vi "ReadWheelVelocity.vi"(8 "error in":errorcluster, 10 "Robot Configuration":T1={"wheel parameters"={"wheel radius"=0.05, "gear ratio"=1.0, "forward rotation direction"=0}, "wheel separation"=0.19, "Encoder Pulse Per Rev"=1856.0, "Update Period (sec)"=0.02, "Initial posture frame"=[0.0, 0.0, 0.0]} {"wheel parameters"."forward rotation direction" items=["Clockwise", "Counterclockwise"]}, 11 "Motor Ref":T4) -> (0 "error out":errorcluster, 2 "Wheel Velocity":T17, 3 "Motor Ref":T4)   [LabVIEW 2016]
uses:
  MotorObject.ctl
  <vilib>/myRIO/Instrument Drivers/Onboard IO/PWM/typedefs/PWM Reference.ctl
  <vilib>/myRIO/Common/Instrument Driver Framework/Utilities/typedefs/myRIO Generic Hardware Reference.ctl
  <vilib>/myRIO/Common/Instrument Driver Framework/Utilities/typedefs/Hardware Version Enum.ctl
  <vilib>/myRIO/Common/Instrument Driver Framework/Utilities/typedefs/myRIO v1.0 Reference.ctl
  <vilib>/myRIO/Common/Instrument Driver Framework/Utilities/typedefs/Generic FPGA Reference.ctl
  <vilib>/myRIO/Common/Instrument Driver Framework/myRIO v1.0/PWM/typedefs/PWM Channels Enum.ctl
  <vilib>/myRIO/Instrument Drivers/Onboard IO/PWM/typedefs/PWM Configuration.ctl
  <vilib>/myRIO/Instrument Drivers/Onboard IO/DIO/typedefs/DIO Reference.ctl
  <vilib>/myRIO/Common/Instrument Driver Framework/myRIO v1.0/DIO/typedefs/DIO Channels List.ctl
  <vilib>/myRIO/Common/Instrument Driver Framework/myRIO v1.0/DIO/typedefs/DIO Channels Enum.ctl
  <vilib>/myRIO/Instrument Drivers/Onboard IO/Encoder/typedefs/Encoder Reference.ctl
  <vilib>/myRIO/Common/Instrument Driver Framework/myRIO v1.0/Encoder/typedefs/Encoder Channels Enum.ctl
  Configurations.ctl
  <vilib>/robotics/Steering/Wheel/Wheel Parameters.ctl
  <vilib>/robotics/Steering/Wheel/Rotation Direction.ctl
  <vilib>/myRIO/Common/Instrument Driver Framework/myRIO v1.0/Encoder/vis/myRIO v1.0 Read Encoder.vi
  <vilib>/myRIO/Common/Instrument Driver Framework/roboRIO v1.0/Encoder/vis/roboRIO v1.0 Read Encoder.vi
  <vilib>/Utility/error.llb/Error Cluster From Error Code.vi
  <vilib>/myRIO/Instrument Drivers/Onboard IO/Encoder/Encoder.lvlib
  <vilib>/myRIO/Instrument Drivers/Onboard IO/DIO/DIO.lvlib
  <vilib>/myRIO/Instrument Drivers/Onboard IO/PWM/PWM.lvlib
  <vilib>/robotics/Steering/Wheel/NI_Robotics_Wheel.lvclass
panel:
  in  "Ref Cluster":T17
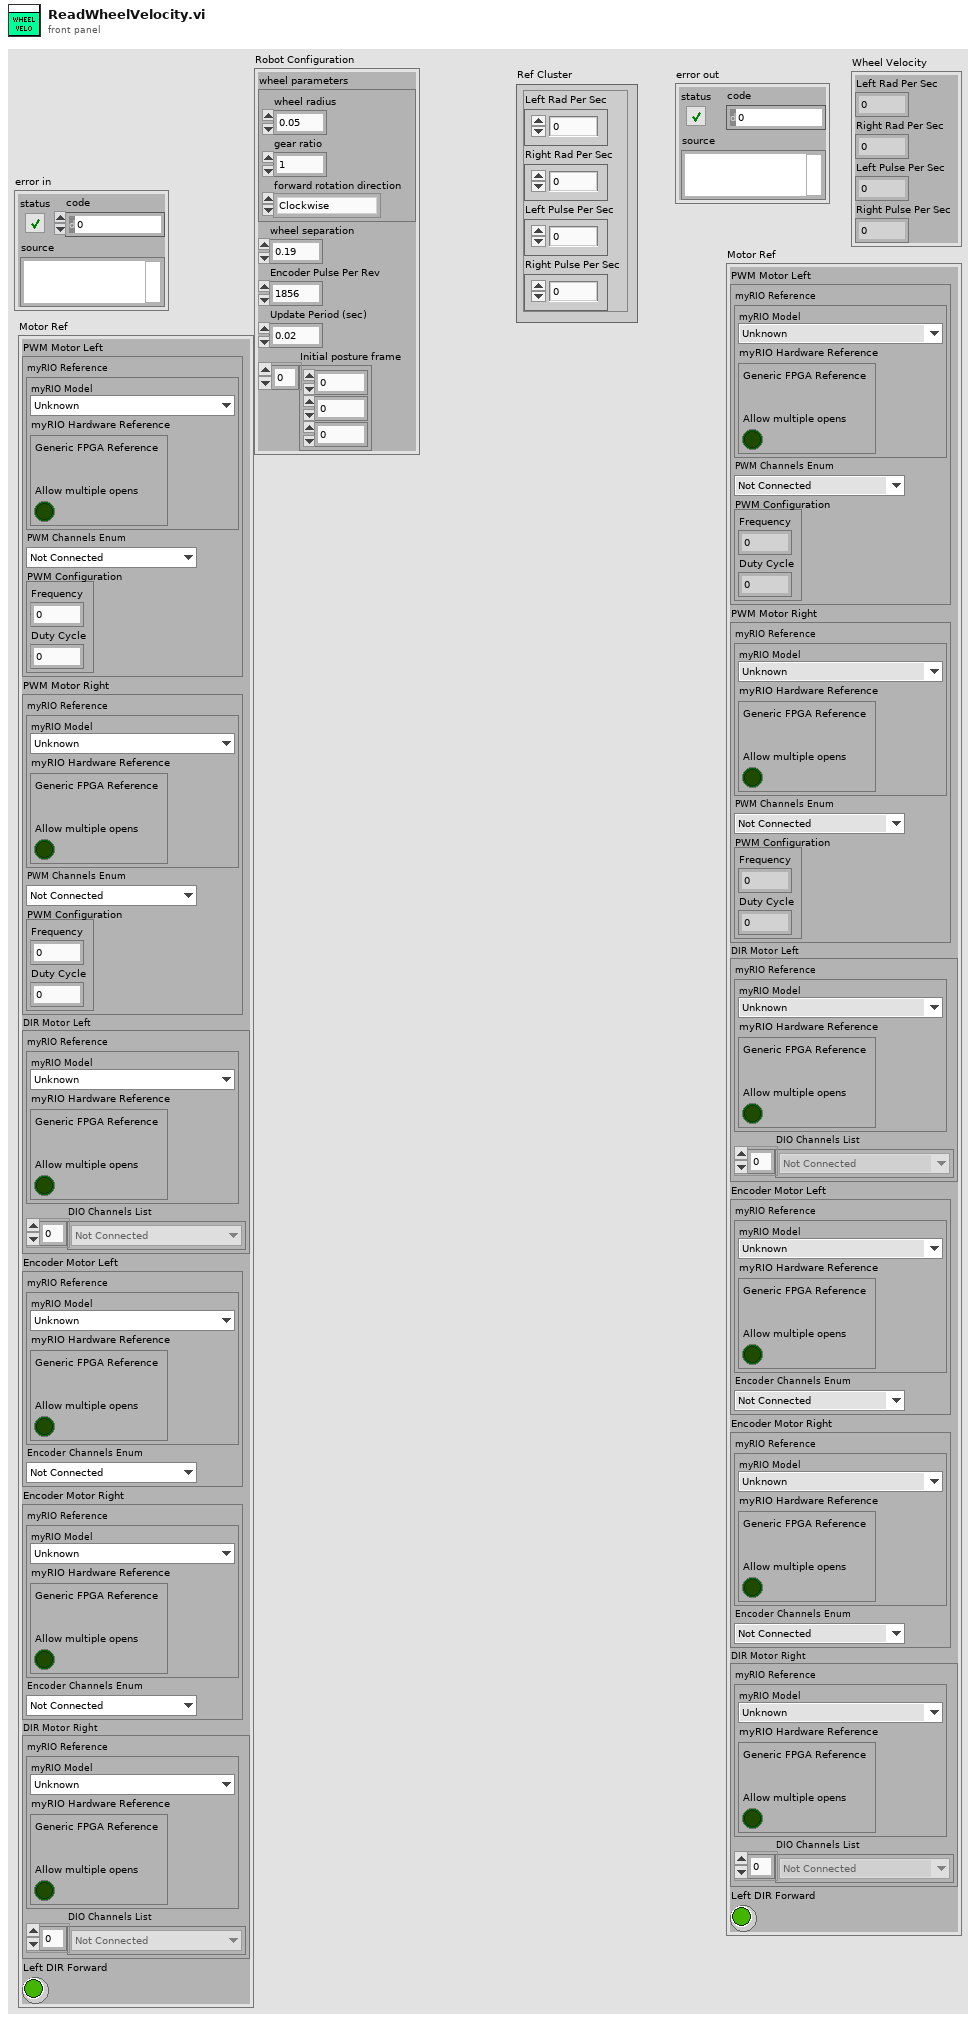
[diagram p1: front panel]
types:
  T1 = typedef "Configurations.ctl" = cluster{"wheel parameters":T2, "wheel separation":dbl, "Encoder Pulse Per Rev":dbl, "Update Period (sec)":dbl, "Initial posture frame":dbl[]}
  T2 = typedef "NI_Robotics_Wheel.lvclass/Wheel Parameters.ctl" = cluster{"wheel radius":dbl, "gear ratio":dbl, "forward rotation direction":T3}
  T3 = typedef "NI_Robotics_Wheel.lvclass/Rotation Direction.ctl" = u16
  T4 = typedef "MotorObject.ctl" = cluster{"PWM Motor Left":T5, "PWM Motor Right":T5, "DIR Motor Left":T12, "Encoder Motor Left":T15, "Encoder Motor Right":T15, "DIR Motor Right":T12, "Left DIR Forward":bool}
  T5 = typedef "PWM.lvlib/PWM Reference.ctl" = cluster{"myRIO Reference":T6, "PWM Channels Enum":T10, "PWM Configuration":T11}
  T6 = typedef "myRIO Generic Hardware Reference.ctl" = cluster{"myRIO Model":T7, "myRIO Hardware Reference":T8}
  T7 = typedef "Hardware Version Enum.ctl" = enum16{"Unknown", "myRIO-1900", "myRIO-1950", "roboRIO", "NI ELVIS RIO CM"}
  T8 = typedef "myRIO v1.0 Reference.ctl" = cluster{"Generic FPGA Reference":T9, "Allow multiple opens":bool}
  T9 = typedef "Generic FPGA Reference.ctl" = refnum<k20>
  T10 = typedef "PWM Channels Enum.ctl" = enum16{"Not Connected", "C/PWM0", "C/PWM1", "A/PWM0", "A/PWM1", "A/PWM2", "B/PWM0", "B/PWM1", "B/PWM2", "PWM/PWM0", "PWM/PWM1", "PWM/PWM2", "PWM/PWM3", "PWM/PWM4", "PWM/PWM5", "PWM/PWM6", "PWM/PWM7", "PWM/PWM8", "PWM/PWM9"}
  T11 = typedef "PWM.lvlib/PWM Configuration.ctl" = cluster{"Frequency":dbl, "Duty Cycle":dbl}
  T12 = typedef "DIO.lvlib/DIO Reference.ctl" = cluster{"myRIO Reference":T6, "DIO Channels List":T13}
  T13 = typedef "DIO Channels List.ctl" = T14[]
  T14 = typedef "DIO Channels Enum.ctl" = enum16{"Not Connected", "C/DIO0", "C/DIO1", "C/DIO2", "C/DIO3", "C/DIO4", "C/DIO5", "C/DIO6", "C/DIO7", "A/DIO0", "A/DIO1", "A/DIO2", "A/DIO3", "A/DIO4", "A/DIO5", "A/DIO6", "A/DIO7", "A/DIO8", "A/DIO9", "A/DIO10", "A/DIO11", "A/DIO12", "A/DIO13", "A/DIO14", "A/DIO15", "B/DIO0", "B/DIO1", "B/DIO2", "B/DIO3", "B/DIO4", "B/DIO5", "B/DIO6", "B/DIO7", "B/DIO8", "B/DIO9", "B/DIO10", "B/DIO11", "B/DIO12", "B/DIO13", "B/DIO14", "B/DIO15", "LED0", "LED1", "LED2", "LED3", "Button0", "DIO/DIO0", "DIO/DIO1", "DIO/DIO2", "DIO/DIO3", "DIO/DIO4", "DIO/DIO5", "DIO/DIO6", "DIO/DIO7", "DIO/DIO8", "DIO/DIO9", "SPI/CS0", "SPI/CS1", "SPI/CS2", "SPI/CS3", "LED RADIO (Green)", "LED RADIO (Red)", "LED COMM (Green)", "LED COMM (Red)", "LED MODE (Green)", "LED MODE (Red)"}
  T15 = typedef "Encoder.lvlib/Encoder Reference.ctl" = cluster{"myRIO Reference":T6, "Encoder Channels Enum":T16}
  T16 = typedef "Encoder Channels Enum.ctl" = enum16{"Not Connected", "C/ENC0", "C/ENC1", "A/ENC", "B/ENC", "DIO/ENC0", "DIO/ENC1", "DIO/ENC2", "DIO/ENC3", "DIO/ENC4"}
  T17 = cluster{"Left Rad Per Sec":dbl, "Right Rad Per Sec":dbl, "Left Pulse Per Sec":dbl, "Right Pulse Per Sec":dbl}
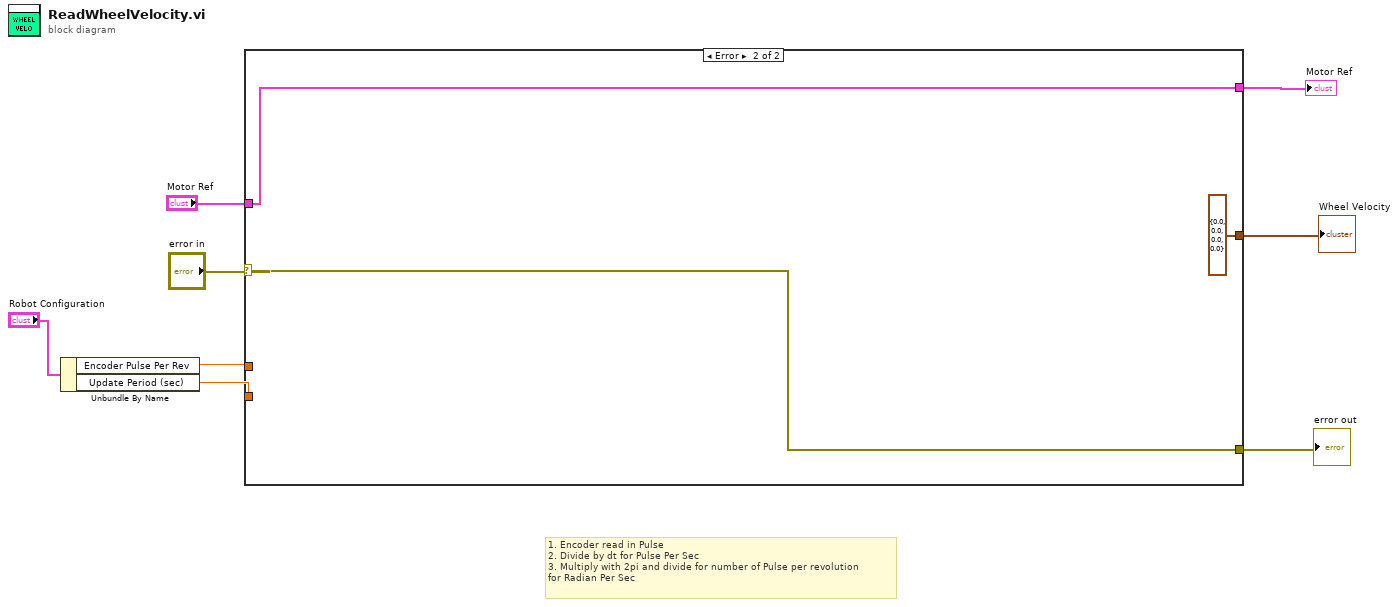
[diagram p0: block diagram]
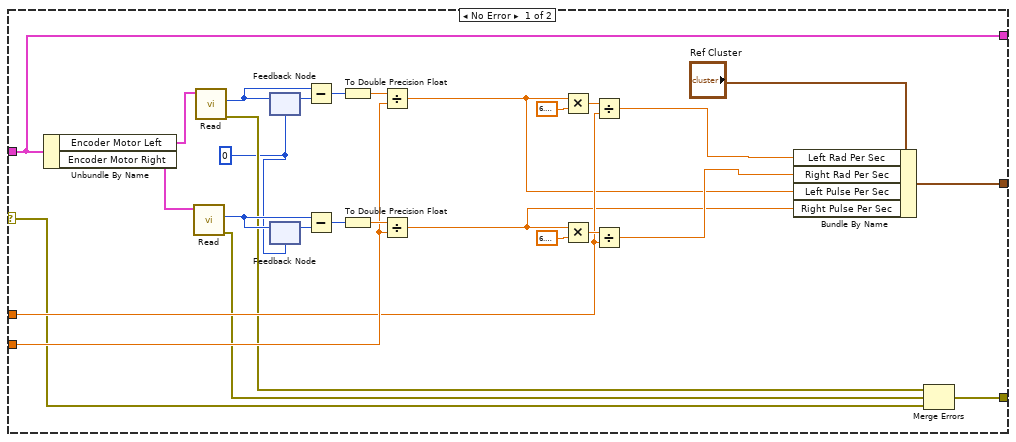
[diagram p2: hidden frame]
diagram:
  # "1. Encoder read in Pulse \n2. Divide by dt for Pulse Per Sec\n3. Multiply with 2pi and divide for number of Pulse per revolution \nfor Radian Per Sec"
  n1 = Unbundle By Name("Robot Configuration") -> ("Encoder Pulse Per Rev"=w2:dbl, "Update Period (sec)"=w1:dbl)
  n2 = case shown="Error" "error in" {
    selector: "error in" -> [w13 w39]
    tunnel: "Motor Ref" -> [w9 w38]
    tunnel: w1 -> [w22 _]
    tunnel: w2 -> [w21 _]
    tunnel: [w12 w39] -> w6
    tunnel: [w11 T17 {"Left Rad Per Sec"=0.0, "Right Rad Per Sec"=0.0, "Left Pulse Per Sec"=0.0, "Right Pulse Per Sec"=0.0} ("Ref Cluster")] -> w5
    tunnel: [w9 w38] -> w4
    frame No Error {
      w10 = 0 ("Counter Value")
      n3 = Unbundle By Name(w9) -> ("Encoder Motor Left"=w27:T15, "Encoder Motor Right"=w28:T15)
      n4 = call <vilib>:"Read.vi"("Encoder Ref In"=w28) -> ("error out"=w14:errorcluster, "Counter Value"=w29:i32)  [unwired: 6 in, 3 out]
      n5 = call <vilib>:"Read.vi"("Encoder Ref In"=w27) -> ("error out"=w15:errorcluster, "Counter Value"=w32:i32)  [unwired: 6 in, 3 out]
      n6 = feedback #1(w10) -> (w31:i32)
      n7 = feedback-in #1(w32) -> ()
      n8 = feedback #2(w10) -> (w30:i32)
      n9 = feedback-in #2(w29) -> ()
      n10 = Subtract(x=w32, y=w31) -> (x-y=w33:i32)
      n11 = Subtract(x=w29, y=w30) -> (x-y=w24:i32)
      n12 = To Double Precision Float(number=w33) -> (double precision float=w34:dbl)
      n13 = To Double Precision Float(number=w24) -> (double precision float=w23:dbl)
      n14 = Divide(x=w34, y=w22) -> (x/y=w17:dbl)
      n15 = Divide(x=w23, y=w22) -> (x/y=w16:dbl)
      n16 = Multiply(x=w17, y=6.283185307179586) -> (x*y=w36:dbl)
      n17 = Multiply(x=w16, y=6.283185307179586) -> (x*y=w26:dbl)
      n18 = Divide(x=w36, y=w21) -> (x/y=w20:dbl)
      n19 = Divide(x=w26, y=w21) -> (x/y=w19:dbl)
      n20 = Bundle By Name(cluster="Ref Cluster", "Left Rad Per Sec"=w20, "Right Rad Per Sec"=w19, "Left Pulse Per Sec"=w17, "Right Pulse Per Sec"=w16) -> (w11:T17)
      n21 = Merge Errors(w15, w14, w13) -> (w12:errorcluster)
    }
    frame Error {
    }
  }
  "error out" <- w6
  "Wheel Velocity" <- w5
  "Motor Ref" <- w4
